vi "ma_get resampling FIR parameters.vi"(9 "filter info":cluster{"h":dbl[], "Max Decimation":dbl}={"h"=[], "Max Decimation"=1024.0} {"Max Decimation" format="%.2f"; "h" format="%.2p"}, 10 "dt":dbl=0.2222222222222222 format="%.2p", 11 "Waveform in":waveform(dbl)={"t0"=timestamp(0 s since 1904-01-01), "dt"=0.001, "Y"=[]}) -> (2 "history size":i32=9742, 3 "Filter parameters":T1 {"half duration" format="%.2f"; "FIR index step" format="%.2f"; "scaled filter" format="%.2p"})   [LabVIEW 2020, in "NI_MAPro.lvlib"]
uses:
  NI_MAPro.lvlib
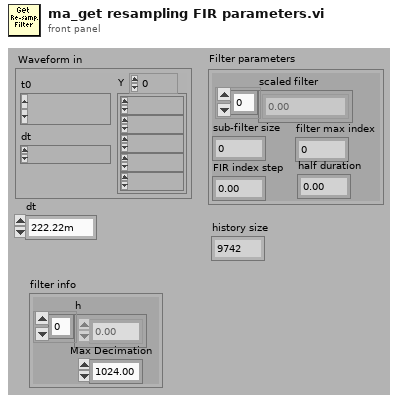
[diagram p1: front panel]
types:
  T1 = cluster{"scaled filter":dbl[], "sub-filter size":i32, "filter max index":i32, "FIR index step":dbl, "half duration":dbl}
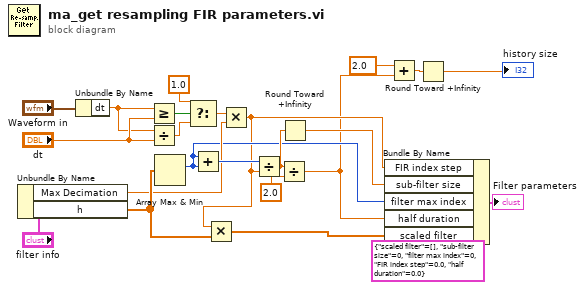
[diagram p0: block diagram]
diagram:
  n1 = Unbundle By Name("filter info") -> ("Max Decimation"=w14:dbl, "h"=w15:dbl[])
  n2 = Unbundle By Name("Waveform in") -> ("dt"=w11:dbl)
  n3 = Greater Or Equal?(x=w11, y="dt") -> (x >= y?=w23:bool)
  n4 = Divide(x=w11, y="dt") -> (x/y=w21:dbl)
  n5 = Array Max & Min(array=w15) -> (max index (indices)=w8:i32)  [unwired: 3 out]
  n6 = Select(t=1.0, s=w23, f=w21) -> (s? t:f=w19:dbl)
  n7 = Add(x=w8, y=w8) -> (x+y=w17:i32)
  n8 = Multiply(x=w19, y=w14) -> (x*y=w6:dbl)
  n9 = Multiply(x=w6, y=w15) -> (x*y=w9:dbl[])
  n10 = Divide(x=w17, y=w6) -> (x/y=w16:dbl)
  n11 = Divide(x=w16, y=2.0) -> (x/y=w4:dbl)
  n12 = Round Toward +Infinity(x=w16) -> (ceil(x): smallest int >= x=w7:dbl)
  n13 = Bundle By Name(cluster=T1 {"scaled filter"=[], "sub-filter size"=0, "filter max index"=0, "FIR index step"=0.0, "half duration"=0.0} ("Filter parameters"), "FIR index step"=w6, "sub-filter size"=w7, "filter max index"=w8, "half duration"=w4, "scaled filter"=w9) -> (→"Filter parameters":T1)
  n14 = Add(x=2.0, y=w4) -> (x+y=w2:dbl)
  n15 = Round Toward +Infinity(x=w2) -> (ceil(x): smallest int >= x=→"history size":dbl)
